vi "init.vi"(8 "error in (no error)":errorcluster, 10 "Resource":string, 11 "FgenKeysight in":refnum<class "ArbKeysight.lvclass">) -> (0 "error out":errorcluster, 3 "FgenKeysight out":refnum<class "ArbKeysight.lvclass">)   [LabVIEW 2023, in "ArbKeysight.lvclass"]
doc: "<b>Author:</b> Wolfgang\n<b>Description:</b> Method to initialize an instrument by resource name (defined in NI MAX) for any instrument category."
uses:
  ArbKeysight.lvclass
  ArbKeysight.lvclass/ArbKeysight.ctl
  Arb.lvclass
  Driver/Keysight-33500B.lvlib
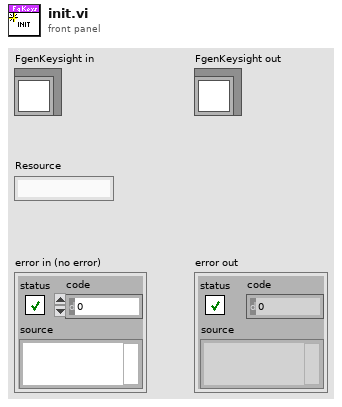
[diagram p1: front panel]
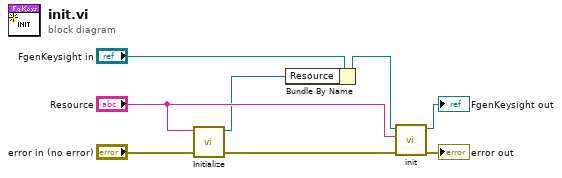
[diagram p0: block diagram]
diagram:
  n1 = call "Initialize.vi"("error in (no error)"="error in (no error)", "VISA resource name"="Resource") -> ("error out"=w3:errorcluster, "VISA resource name out"=w1:refnum<visa-resource-name>)  [unwired: 8 in]
  n2 = Bundle By Name(cluster="FgenKeysight in", "Resource"=w1) -> (w2:refnum<class "ArbKeysight.lvclass">)
  n3 = call-parent "init.vi"("error in (no error)"=w3, "Resource"="Resource", "Instrument in"=w2) -> ("error out"=→"error out":errorcluster, "Instrument out"=→"FgenKeysight out":refnum<class "ArbKeysight.lvclass">)  [unwired: 7 in]
